vi "Pythagorean Theorem.vi"(10 "B":dbl, 11 "A":dbl) -> (3 "C":dbl)   [LabVIEW 2014]
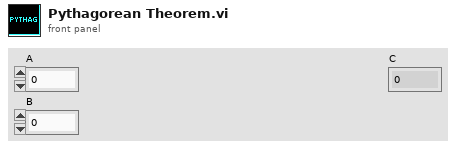
[diagram p1: front panel]
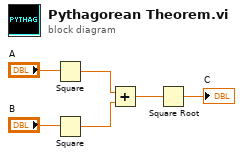
[diagram p0: block diagram]
diagram:
  n1 = Square(x="A") -> (x^2=w5:dbl)
  n2 = Square(x="B") -> (x^2=w4:dbl)
  n3 = Add(x=w5, y=w4) -> (x+y=w6:dbl)
  n4 = Square Root(x=w6) -> (sqrt(x)=→"C":dbl)
